vi "Begin.vi"() -> (0 "Initialiser":bool)   [LabVIEW 2014]
doc: "Called before other user functions, this VI is expected to open initial I/O refnums, load in file data, and do all program initialization. Notice that the <B>error out</B> terminal is simply used for data flow. Wiring it to other structures or subVIs ensures that this VI runs first."
uses:
  <vilib>/Rock Robotics/WPI/DriverStation/WPI_DriverStationRobotMode2.ctl
  Robot Global Data.vi
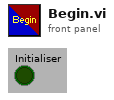
[diagram p1: front panel]
types:
  T1 = typedef "WPI_DriverStationRobotMode2.ctl" = enum16{"Autonomous Disabled", "Autonomous Enabled", "Teleop Disabled", "Teleop Enabled", "Disconnected", "Finish", "Test Disabled", "Test Enabled"}
  T2 = enum16{"Nothing", "Load", "Lock", "Pass", "Grab", "Loader Down", "Shoot", "Auto Start", "Tele Start"}
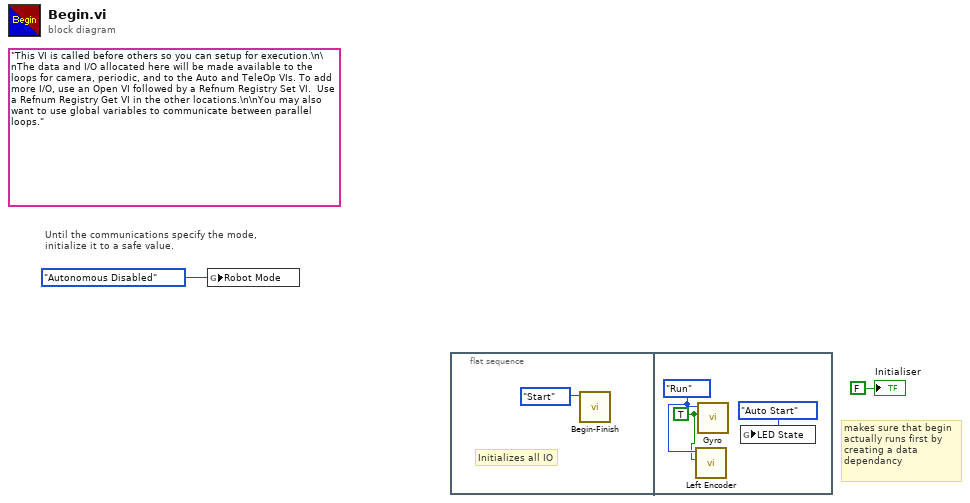
[diagram p0: block diagram]
diagram:
  (unwired) "This VI is called before others so you can setup for execution.\n\nThe data and I/O allocated here will be made available to the loops for camera, periodic, and to the Auto and TeleOp VIs. To add more I/O, use an Open VI followed by a Refnum Registry Set VI.  Use a Refnum Registry Get VI in the other locations.\n\nYou may also want to use global variables to communicate between parallel loops."
  # "makes sure that begin\nactually runs first by\ncreating a data \ndependancy"
  # "Until the communications specify the mode,\ninitialize it to a safe value."
  n1 = global write "Robot Global Data.vi" "Robot Mode"(WPI_DriverStationRobotMode2."Autonomous Disabled" ("Robot Mode")) -> ()
  n2 = flat-sequence {
    frame #0 {
      # "Initializes all IO"
      n3 = call "Begin-Finish.vi"("Enum"=enum16{"Start", "Run", "End"}."Start") -> ()  [unwired: 11 in]
    }
    frame #1 {
      w6 = enum16{"Start", "Run", "End"}."Run" ("Enum")
      w5 = TRUE ("Reset")
      n4 = call "Left Encoder.vi"("Reset"=w5, "Enum"=w6) -> ()  [unwired: 8 in, 2 out]
      n5 = call "Gyro.vi"("Reset"=w5, "Enum"=w6) -> ()  [unwired: 9 in, 1 out]
      n6 = global write "Robot Global Data.vi" "LED State"(T2."Auto Start" ("LED State")) -> ()
    }
  }
  "Initialiser" <- FALSE
